vi "3.vi"() -> ()   [LabVIEW 2023]
uses:
  <vilib>/Analysis/8numeric.llb/1D Numeric Integration.vi
  <vilib>/Analysis/NI_AALPro.lvlib
panel:
  in  "stop":bool
  out "Arie":dbl
  out "yV":dbl
  out "xV":dbl
  out "x2 c":cdb
  out "x1 c":cdb
  out "x 2":dbl
  out "x1":dbl
  in  "Nr puncte grafic":u16
  in  "c":dbl(slide) scale=-10.0..10.0
  in  "b":dbl(slide) scale=-10.0..10.0
  in  "a":dbl(slide) scale=-10.0..10.0
  in  "x min - x max":cluster{dbl, dbl}(slide) scale=-10.0..10.0
  out "XY Graph":cluster{dbl[], dbl[]}(graph)
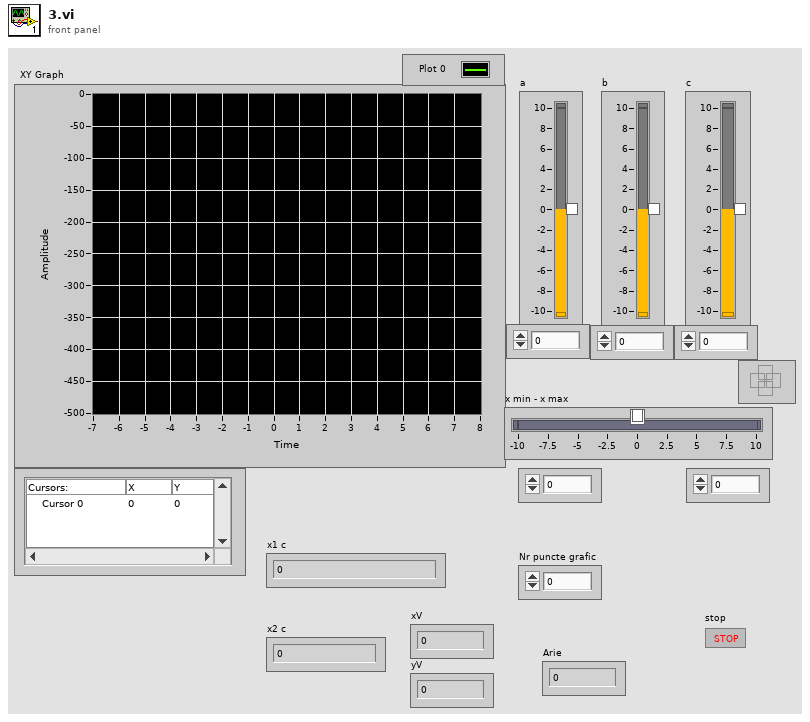
[diagram p1: front panel]
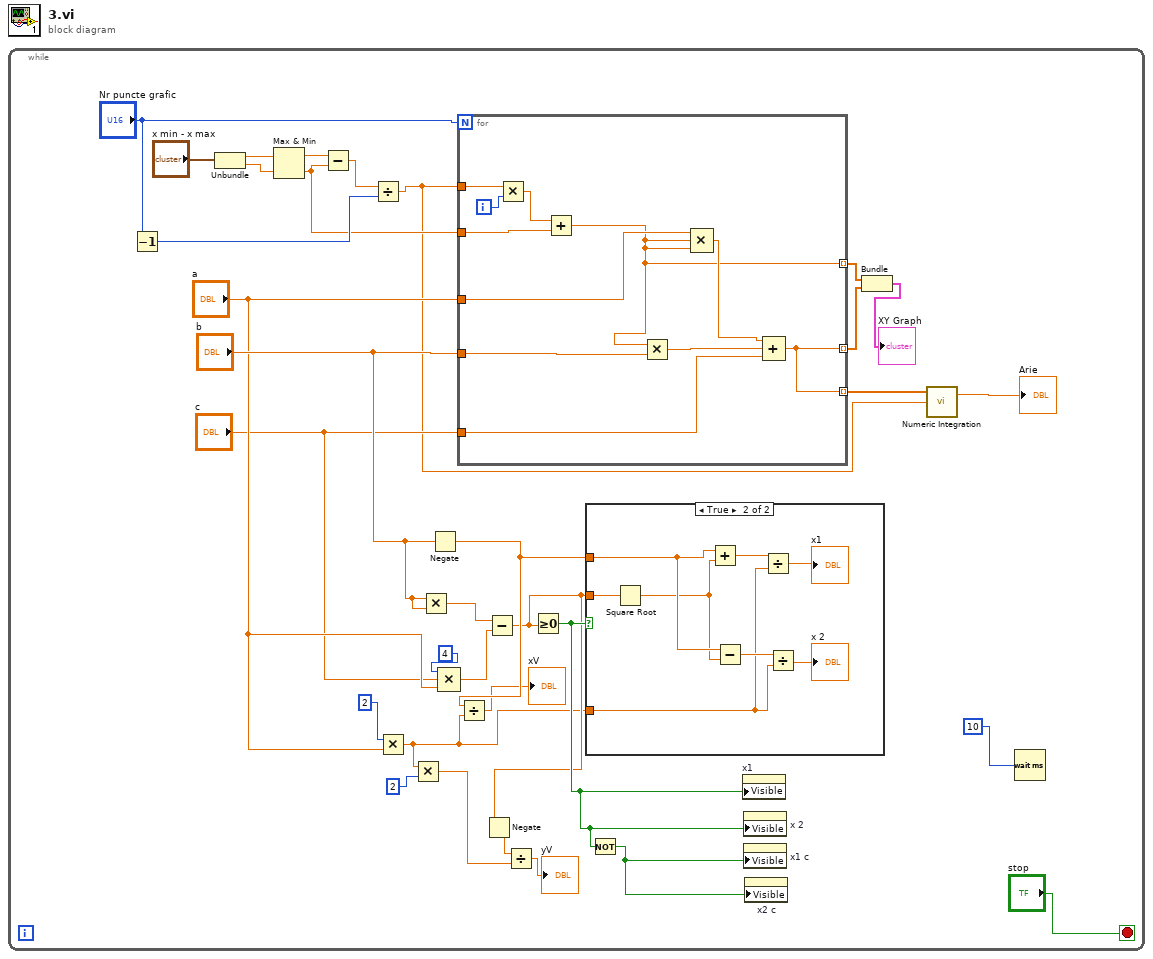
[diagram p0: block diagram]
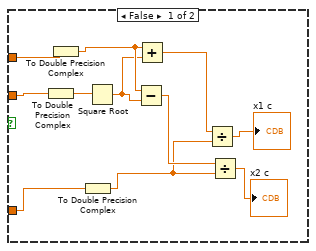
[diagram p2: hidden frame]
diagram:
  n1 = while {
    stop <- "stop" stop-if-true
    n2 = Decrement(x="Nr puncte grafic") -> (x-1=w27:u16)
    n3 = Unbundle("x min - x max") -> (w31:dbl, w30:dbl)
    n4 = Max & Min(x=w31, y=w30) -> (max(x,y)=w29:dbl, min(x,y)=w26:dbl)
    n5 = Subtract(x=w29, y=w26) -> (x-y=w28:dbl)
    n6 = Divide(x=w28, y=w27) -> (x/y=w4:dbl)
    n7 = Multiply(x=2, y="a") -> (x*y=w10:dbl)
    n8 = Multiply(x=w10, y=2) -> (x*y=w7:dbl)
    n9 = Multiply(x="b", y="b") -> (x*y=w21:dbl)
    n10 = Negate(x="b") -> (-x=w13:dbl)
    n11 = Compound Arithmetic op=MULTIPLY(4, "c", "a") -> (w19:dbl)
    n12 = for {
      N: "Nr puncte grafic" -> [_]
      tunnel: "c" -> [w60]
      tunnel: "b" -> [w59]
      tunnel: w26 -> [w58]
      tunnel: w4 -> [w56]
      tunnel: "a" -> [w55]
      tunnel: [w53] -> w25 mode=indexing
      tunnel: [w54] -> w24 mode=indexing
      tunnel: [w53] -> w5 mode=indexing
      i -> [w57]
      n13 = Multiply(x=w56, y=w57) -> (x*y=w63:dbl)
      n14 = Add(x=w63, y=w58) -> (x+y=w54:dbl)
      n15 = Multiply(x=w54, y=w59) -> (x*y=w61:dbl)
      n16 = Compound Arithmetic op=MULTIPLY(w55, w54, w54) -> (w62:dbl)
      n17 = Compound Arithmetic op=ADD(w62, w61, w60) -> (w53:dbl)
    }
    n18 = Divide(x=w13, y=w10) -> (x/y=→"xV":dbl)
    n19 = Subtract(x=w21, y=w19) -> (x-y=w11:dbl)
    n20 = Negate(x=w11) -> (-x=w8:dbl)
    n21 = Divide(x=w8, y=w7) -> (x/y=→"yV":dbl)
    n22 = Greater Or Equal To 0?(x=w11) -> (x >= 0?=w15:bool)
    n23 = case shown="True" w15 {
      tunnel: w13 -> [w44 w48]
      tunnel: w10 -> [w42 w47]
      tunnel: w11 -> [w43 w45]
      frame False {
        n24 = To Double Precision Complex(1:w43) -> (0:w41:cdb)
        n25 = To Double Precision Complex(1:w44) -> (0:w40:cdb)
        n26 = To Double Precision Complex(1:w42) -> (0:w36:cdb)
        n27 = Square Root(x=w41) -> (sqrt(x)=w39:cdb)
        n28 = Subtract(x=w40, y=w39) -> (x-y=w37:cdb)
        n29 = Add(x=w40, y=w39) -> (x+y=w38:cdb)
        n30 = Divide(x=w38, y=w36) -> (x/y=→"x1 c":cdb)
        n31 = Divide(x=w37, y=w36) -> (x/y=→"x2 c":cdb)
      }
      frame True {
        n32 = Square Root(x=w45) -> (sqrt(x)=w46:dbl)
        n33 = Add(x=w48, y=w46) -> (x+y=w50:dbl)
        n34 = Subtract(x=w48, y=w46) -> (x-y=w49:dbl)
        n35 = Divide(x=w50, y=w47) -> (x/y=→"x1":dbl)
        n36 = Divide(x=w49, y=w47) -> (x/y=→"x 2":dbl)
      }
    }
    n37 = Not(x=w15) -> (.not. x?=w14:bool)
    n38 = property on="x1" class="DigNum (strict)"("Visible"=w15) -> ()  [unwired: 2 in, 2 out]
    n39 = property on="x 2" class="DigNum (strict)"("Visible"=w15) -> ()  [unwired: 2 in, 2 out]
    n40 = property on="x1 c" class="DigNum (strict)"("Visible"=w14) -> ()  [unwired: 2 in, 2 out]
    n41 = property on="x2 c" class="DigNum (strict)"("Visible"=w14) -> ()  [unwired: 2 in, 2 out]
    n42 = Bundle(w24, w25) -> (→"XY Graph":cluster{dbl[], dbl[]})  [unwired: 1 in]
    n43 = call-poly <vilib>:"Numeric Integration.vi"("dt"=w4, "Input Array"=w5) -> ("result"=→"Arie":dbl)  [unwired: 1 in, 1 out]
    n44 = Wait (ms)(milliseconds to wait=10) -> ()  [unwired: 1 out]
  }
